vi "调整主控件尺寸.vi"() -> ()   [LabVIEW 2010]
doc: "本VI是为《我和LabVIEW》一书编写的示例。\n关于本书的介绍请参考网页：\nhttp://ruanqizhen.spaces.live.com/blog/cns!5852D4F797C53FB6!4310.entry"
panel:
  out "Waveform Chart":dbl(graph)
  out "波形图":dbl[](graph)
  in  "停止 2":bool
  in  "停止":bool
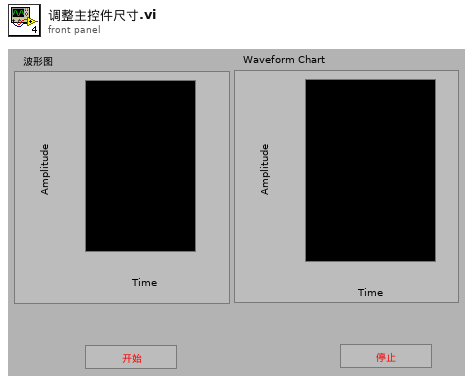
[diagram p1: front panel]
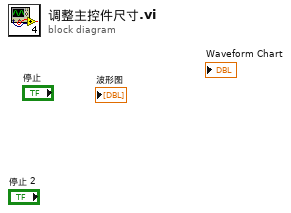
[diagram p0: block diagram]
diagram:
